vi "calc_angles.vi"(2 "lines/mm":dbl, 3 "Central Wavlength (nm)":dbl) -> (0 "camera angle":dbl, 1 "grating angle":dbl)   [LabVIEW 2015]
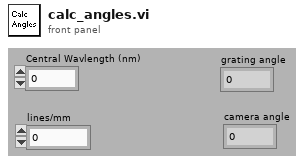
[diagram p1: front panel]
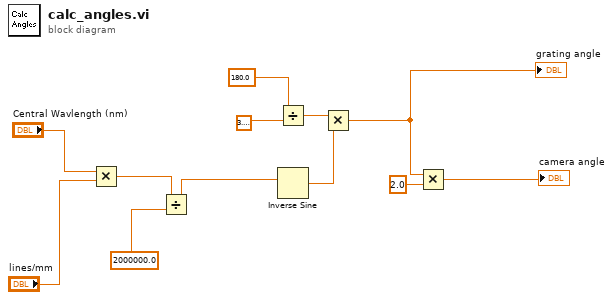
[diagram p0: block diagram]
diagram:
  n1 = Multiply(x="Central Wavlength (nm)", y="lines/mm") -> (x*y=w5:dbl)
  n2 = Divide(x=w5, y=2000000.0) -> (x/y=w4:dbl)
  n3 = Divide(x=180.0 ("y"), y=3.141592653589793) -> (x/y=w12:dbl)
  n4 = Inverse Sine(1:w4) -> (0:w11:dbl)
  n5 = Multiply(x=w12, y=w11) -> (x*y=w10:dbl)
  "grating angle" <- w10
  n6 = Multiply(x=w10, y=2.0) -> (x*y=→"camera angle":dbl)
